vi "Read Name.vi"(11 "Proccess in":refnum<class "Proccess.lvclass">) -> (1 "ParentName":string, 2 "Name":string)   [LabVIEW 2019, in "Proccess.lvclass"]
uses:
  Proccess.lvclass
  Proccess.lvclass/Proccess.ctl
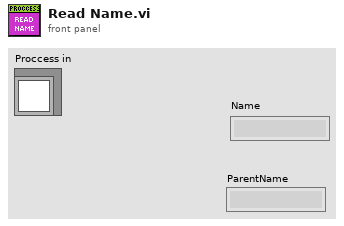
[diagram p1: front panel]
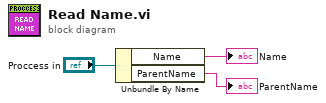
[diagram p0: block diagram]
diagram:
  n1 = Unbundle By Name("Proccess in") -> ("Name"=→"Name":string, "ParentName"=→"ParentName":string)
